vi "Generate Command Frame Vectors.vi"(0 "RFFE Standard Command in":refnum<class "RFFE Standard Command.lvclass">, 11 "error in (no error)":errorcluster) -> (4 "RFFE Standard Command out":refnum<class "RFFE Standard Command.lvclass">, 6 "Command Frame Vectors":string[](array[string]), 15 "error out":errorcluster)   [LabVIEW 2018, in "MIPI RFFE API.lvlib" / "RFFE Standard Command.lvclass"]
uses:
  RFFE Standard Command.lvclass
  C:/Users/semoore/Projects/mipi-rffe-labview-oop/Command/RFFE Command.lvclass
  Command/Get Slave Address Field Width.vi
  Command/RFFE Command.lvclass
  MIPI RFFE API.lvlib
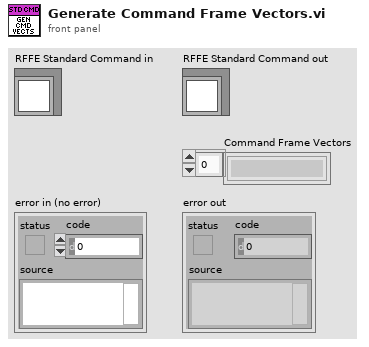
[diagram p1: front panel]
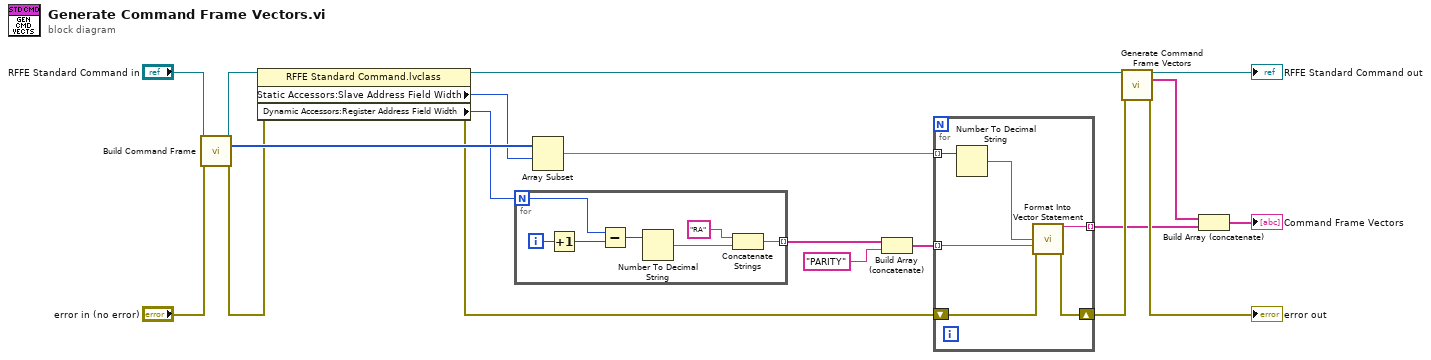
[diagram p0: block diagram]
diagram:
  n1 = call-dynamic "Build Command Frame.vi"("RFFE Standard Command in"="RFFE Standard Command in", "error in (no error)"="error in (no error)") -> ("RFFE Standard Command out"=w16:refnum<class "RFFE Standard Command.lvclass">, "Command Frame"=w15:u8[], "error out"=w11:errorcluster)  [unwired: 11 in]
  n2 = property class="RFFE Standard Command.lvclass"(reference=w16, error in=w11) -> (reference out=w18:refnum<class "RFFE Standard Command.lvclass">, error out=w2:errorcluster, "Static Accessors:Slave Address Field Width"=w14:i32, "Dynamic Accessors:Register Address Field Width"=w12:i32)
  n3 = for {
    N: w12 -> [w24]
    tunnel: [w20] -> w8 mode=indexing
    i -> [w26]
    n4 = Increment(x=w26) -> (x+1=w25:i32)
    n5 = Subtract(x=w24, y=w25) -> (x-y=w23:i32)
    n6 = Number To Decimal String(number=w23) -> (decimal integer string=w22:string)  [unwired: 1 in]
    n7 = Concatenate Strings("RA", w22) -> (w20:string)
  }
  n8 = Array Subset(array=w15, index=w14) -> (w5:u8[])  [unwired: 1 in]
  n9 = Build Array (concatenate)(w8, "PARITY" ("format string")) -> (w6:string[])
  n10 = for {
    tunnel: w6 -> [w32] mode=indexing
    tunnel: w5 -> [w31] mode=indexing
    shift-right: [w30] -> w3
    shift-left: w2 -> [w29]
    tunnel: [w28] -> w1 mode=indexing
    n11 = Number To Decimal String(number=w31) -> (decimal integer string=w27:string)  [unwired: 1 in]
    n12 = call "Format Into Vector Statement.vi"("DATA (0)"=w27, "Comment"=w32, "error in (no error)"=w29) -> ("Vector Statement"=w28:string, "error out"=w30:errorcluster)  [unwired: 11 in]
  }
  n13 = call-parent "Generate Command Frame Vectors.vi"("RFFE Command in"=w18, "error in (no error)"=w3) -> ("RFFE Command out"=→"RFFE Standard Command out":refnum<class "RFFE Standard Command.lvclass">, "Command Frame Vectors"=w10:string[], "error out"=→"error out":errorcluster)  [unwired: 11 in]
  n14 = Build Array (concatenate)(w10, w1) -> (→"Command Frame Vectors":string[])
